vi "Compute Deconvolved IRF Plot.vi"(4 "# Fit Plot Points":i32=65536, 6 "IRF*PSED fixed Parameters":T1={"order"=0, "T"=0.0, "Time Constant Array"=[], "{S_k, C_k, phi_k, e_k} arrays"={"S_k Array"=[], "C_k Array"=[], "phi_k Array"=[], "e_k Array"=[]}, "IRF Extraction Options"={"Time Constant for IRF Extraction"=1e-18, "IRF Order"=0, "Fourier Series Smoothing"=enum."None", "Noise Threshold"=0.0, "Smoothing Width"=0.0, "Fourier Series Truncation"=enum."Automatic", "Truncation Order"=0, "Save Power Spectrum"=FALSE, "Smoothing"=FALSE, "Smoothing Parameter"=0.0, "Smoothing Order"=1, "Method"=enum."Direct"}} {"IRF Extraction Options"."Smoothing Order" min=1 max=10; "IRF Extraction Options"."Time Constant for IRF Extraction" format="%#_5g"}, 7 "XYGraph in":T6, 8 "error in (no error)":errorcluster, 9 "Fit Parameter Values":dbl[](array[numeric]), 10 "Plot Name":string, 11 "Fitted Decay":cluster{"X Array":dbl[], "Y Array":dbl[]}) -> (0 "error out":errorcluster, 1 "Amplitude String":string, 2 "Power Spectrum":dbl[](array[numeric]), 3 "IRF Plot":cluster{"X Array":dbl[], "Y Array":dbl[]}, 5 "Smoothed Power Spectrum":dbl[](array[numeric]))   [LabVIEW 2021, in "Fits.lvlib"]
uses:
  Fits.lvlib
  Graphs/XY Graph/XY Graph Refnum.ctl
  IRF(X)PSED Fixed Parameters v3.ctl
  IRF(X)PSED Extraction Options.ctl
  Fourier Series Smoothing Option.ctl
  Fourier Series Truncation.ctl
  IRF Extraction Method.ctl
  908e9038-7821-4251-955b-b37bdb3470f5.vi
  IRF Options.vi
  Graphs/XY Graph/XY Graph Add Single Plot with Name.vi
  Graphs/XY Graph/XY Graph Add-Ons.lvlib
  Arrays/Arrays.lvlib
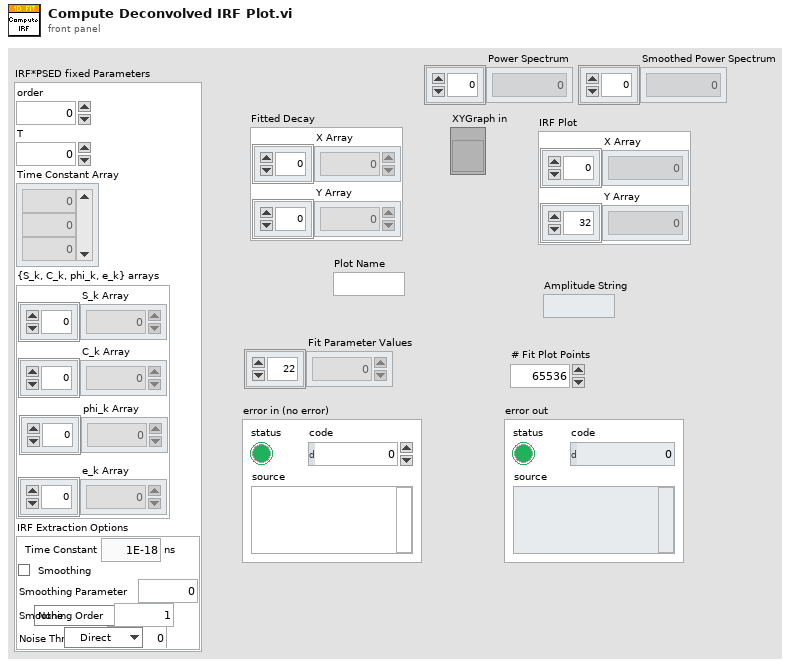
[diagram p1: front panel]
types:
  T1 = typedef "Fits.lvlib/IRF(X)PSED Fixed Parameters v3.ctl" = cluster{"order":i32, "T":dbl, "Time Constant Array":dbl[], "{S_k, C_k, phi_k, e_k} arrays":cluster{"S_k Array":dbl[], "C_k Array":dbl[], "phi_k Array":dbl[], "e_k Array":dbl[]}, "IRF Extraction Options":T2}
  T2 = typedef "Fits.lvlib/IRF(X)PSED Extraction Options.ctl" = cluster{"Time Constant for IRF Extraction":dbl[unit], "IRF Order":i32, "Fourier Series Smoothing":T3, "Noise Threshold":dbl, "Smoothing Width":dbl, "Fourier Series Truncation":T4, "Truncation Order":i32, "Save Power Spectrum":bool, "Smoothing":bool, "Smoothing Parameter":dbl, "Smoothing Order":u32, "Method":T5}
  T3 = typedef "Fits.lvlib/Fourier Series Smoothing Option.ctl" = enum16{"None", "Lanczos Factors", "Fejer Summation"}
  T4 = typedef "Fits.lvlib/Fourier Series Truncation.ctl" = enum16{"Automatic", "Fixed"}
  T5 = typedef "Fits.lvlib/IRF Extraction Method.ctl" = enum16{"Direct", "Topless", "Toeplitz"}
  T6 = typedef "XY Graph Add-Ons.lvlib/XY Graph Refnum.ctl" = refnum<vi>
  T7 = enum16{"Sum of Exponentials", "Squared Sum of Exponentials", "Fourier Series"}
  T8 = typedef "XY Graph Add-Ons.lvlib/XY Plot Data.ctl" = cluster{"X Array":dbl[], "Y Array":dbl[]}
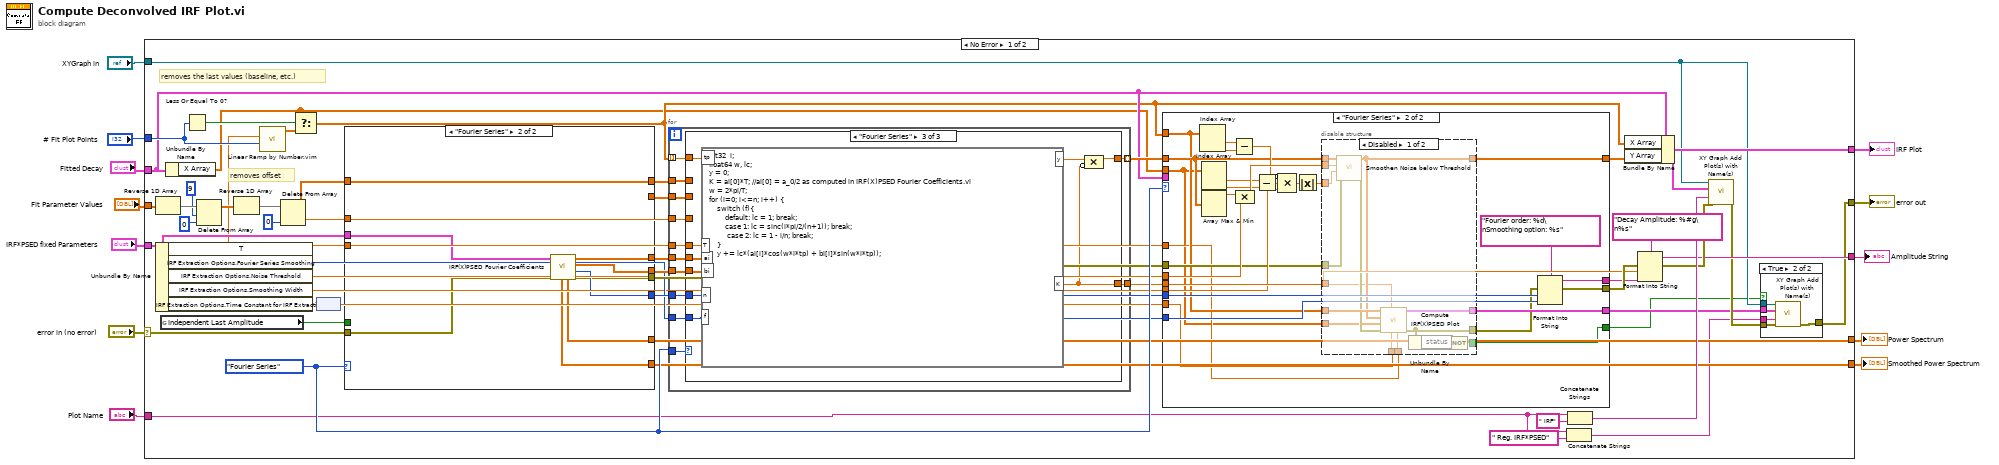
[diagram p0: block diagram]
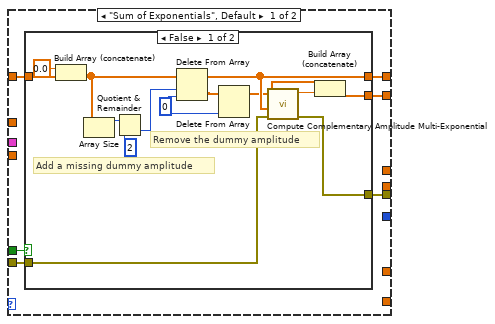
[diagram p5: hidden frame]
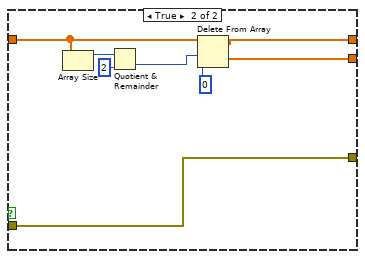
[diagram p6: hidden frame]
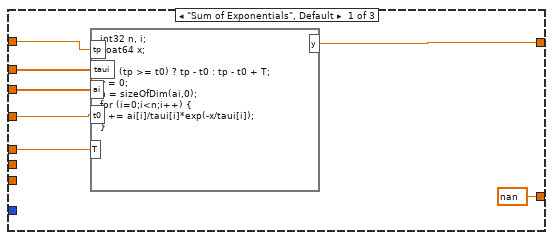
[diagram p7: hidden frame]
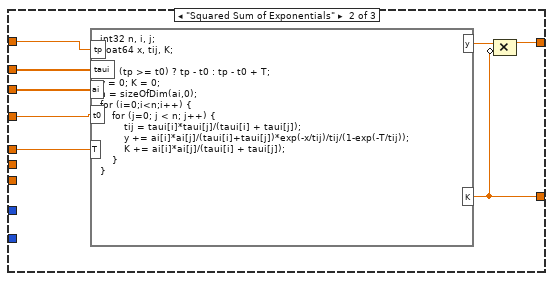
[diagram p8: hidden frame]
diagram:
  n1 = case shown="No Error" "error in (no error)" {
    selector: "error in (no error)" -> [w34 w191]
    tunnel: "Fit Parameter Values" -> [w60 _]
    tunnel: "Fitted Decay" -> [w37 _]
    tunnel: [w63 _] -> w10
    tunnel: "XYGraph in" -> [w21 _]
    tunnel: [w19 w191] -> w8
    tunnel: "IRF*PSED fixed Parameters" -> [w44 _]
    tunnel: "Plot Name" -> [w16 _]
    tunnel: "# Fit Plot Points" -> [w52 _]
    tunnel: [w48 _] -> w4
    tunnel: [w27 _] -> w2
    tunnel: [w26 _] -> w1
    frame No Error {
      w40 = T7."Fourier Series" ("IRF Model")
      # "removes offset"
      # "removes the last values (baseline, etc.)"
      n2 = Reverse 1D Array(array=w60) -> (reversed array=w59:dbl[])
      n3 = Unbundle By Name(w44) -> ("T"=w23:dbl, "IRF Extraction Options.Fourier Series Smoothing"=w30:T3, "IRF Extraction Options.Noise Threshold"=w28:dbl, "IRF Extraction Options.Smoothing Width"=w29:dbl, "IRF Extraction Options.Time Constant for IRF Extraction"=w24:dbl[unit])
      n4 = global read "IRF Options.vi" "Independent Last Amplitude"() -> (w45:bool)
      n5 = Unbundle By Name(w37) -> ("X Array"=w25:dbl[])
      n6 = Less Or Equal To 0?(x=w52) -> (x <= 0?=w53:bool)
      n7 = Delete From Array(array=w59, length=9, index=0) -> (array with subset deleted=w58:dbl[])  [unwired: 1 out]
      n8 = Reverse 1D Array(array=w58) -> (reversed array=w55:dbl[])
      n9 = call "Linear Ramp by Number.vim"("# Steps (1)"=w52, "End (1)"=w23) -> ("Ramp"=w51:dbl[])  [unwired: 7 in, 2 out]
      n10 = Delete From Array(array=w55, index=0) -> (deleted portion=w43:dbl, array with subset deleted=w54:dbl[])  [unwired: 1 in]
      n11 = Select(t=w25, s=w53, f=w51) -> (s? t:f=w36:dbl[])
      n12 = node(w24) -> (w22:dbl)
      n13 = case shown="\"Fourier Series\"" w40 {
        tunnel: w54 -> [w123 w154]
        tunnel: [w122 w154] -> w47
        tunnel: [w121 _] -> w46
        tunnel: w45 -> [w120 _]
        tunnel: w44 -> [_ w151]
        tunnel: w43 -> [_ _]
        tunnel: w23 -> [_ _]
        tunnel: [_ w153] -> w42
        tunnel: [_ w152] -> w41
        tunnel: [_ w150] -> w35
        tunnel: w34 -> [w119 w149]
        tunnel: [w118 w148] -> w33
        tunnel: [_ w147] -> w27
        tunnel: [_ w146] -> w26
        frame "Sum of Exponentials", Default {
          n14 = case shown="False" w120 {
            tunnel: w123 -> [w137 w141]
            tunnel: [w133 w140] -> w122
            tunnel: [w130 w139] -> w121
            tunnel: w119 -> [w125 w138]
            tunnel: [w124 w138] -> w118
            frame False {
              w134 = 0 ("index")
              # "Remove the dummy amplitude"
              # "Add a missing dummy amplitude"
              n15 = Build Array (concatenate)(0.0 ("element"), w137) -> (w127:dbl[])
              n16 = Array Size(array=w127) -> (size(s)=w128:i32)
              n17 = Quotient & Remainder(x=w128, y=2) -> (floor(x/y)=w126:i32)  [unwired: 1 out]
              n18 = Delete From Array(array=w127, length=w126, index=w134) -> (deleted portion=w135:dbl[], array with subset deleted=w133:dbl[])
              n19 = Delete From Array(array=w135, index=w134) -> (array with subset deleted=w132:dbl[])  [unwired: 1 in, 1 out]
              n20 = call "Compute Complementary Amplitude Multi-Exponential.vi"("Error In"=w125, "Time Constant Array"=w133, "Amplitude Array"=w132) -> ("Error Out"=w124:errorcluster, "Complementary Amplitude"=w131:dbl)  [unwired: 7 in]
              n21 = Build Array (concatenate)(w132, w131) -> (w130:dbl[])
            }
            frame True {
              n22 = Array Size(array=w141) -> (size(s)=w143:i32)
              n23 = Quotient & Remainder(x=w143, y=2) -> (floor(x/y)=w142:i32)  [unwired: 1 out]
              n24 = Delete From Array(array=w141, length=w142, index=0) -> (deleted portion=w139:dbl[], array with subset deleted=w140:dbl[])
            }
          }
        }
        frame "Fourier Series" {
          n25 = call "IRF(X)PSED Fourier Coefficients.vi"("Error In"=w149, "IRF*PSED fixed Parameters"=w151) -> ("Error Out"=w148:errorcluster, "Optimal Order"=w150:i32, "[b_k]"=w152:dbl[], "[a_k]"=w153:dbl[], "[s_k]"=w147:dbl[], "Smoothed [s_k]"=w146:dbl[])  [unwired: 4 in]
        }
      }
      n26 = for {
        tunnel: w36 -> [w166] mode=indexing
        tunnel: w43 -> [w165]
        tunnel: w46 -> [w164]
        tunnel: w47 -> [w163]
        tunnel: [w162] -> w39 mode=indexing
        tunnel: w23 -> [w161]
        tunnel: [w160] -> w13
        tunnel: w40 -> [w159]
        tunnel: w42 -> [w158]
        tunnel: w41 -> [w157]
        tunnel: w30 -> [w155]
        tunnel: w35 -> [w156]
        n27 = case shown="\"Fourier Series\"" w159 {
          tunnel: w166 -> [w173 w181 w190]
          tunnel: w165 -> [w172 w180 _]
          tunnel: w164 -> [w171 w179 _]
          tunnel: w163 -> [w170 w178 _]
          tunnel: [w169 w175 w187] -> w162
          tunnel: w161 -> [w168 w176 w188]
          tunnel: [nan ("K") w174 w186] -> w160
          tunnel: w158 -> [_ _ w185]
          tunnel: w157 -> [_ _ w182]
          tunnel: w156 -> [_ _ w184]
          tunnel: w155 -> [_ _ w183]
          frame "Sum of Exponentials", Default {
            n28 = formula code="int32 n, i;\nfloat64 x;\n\nx = (tp >= t0) ? tp - t0 : tp - t0 + T;\ny = 0;\nn = sizeOfDim(ai,0);\nfor (i=0;i<n;i++) {\ny += ai[i]/taui[i]*exp(-x/taui[i]);\n}"("tp"=w173, "t0"=w172, "ai"=w171, "taui"=w170, "T"=w168) -> ("y"=w169:dbl)
          }
          frame "Squared Sum of Exponentials" {
            n29 = formula code="int32 n, i, j;\nfloat64 x, tij, K;\n\nx = (tp >= t0) ? tp - t0 : tp - t0 + T;\ny = 0; K = 0;\nn = sizeOfDim(ai,0);\nfor (i=0;i<n;i++) {\n    for (j=0; j < n; j++) {\n        tij = taui[i]*taui[j]/(taui[i] + taui[j]);\n        y += ai[i]*ai[j]/(taui[i]+taui[j])*exp(-x/tij)/tij/(1-exp(-T/tij));\n        K += ai[i]*ai[j]/(taui[i] + taui[j]);\n    }\n}"("tp"=w181, "t0"=w180, "ai"=w179, "taui"=w178, "T"=w176) -> ("y"=w177:dbl, "K"=w174:dbl)
            n30 = Compound Arithmetic op=MULTIPLY(w177, invert w174) -> (w175:dbl)
          }
          frame "Fourier Series" {
            n31 = formula code="int32  i;\nfloat64 w, lc;\ny = 0;\nK = ai[0]*T; //ai[0] = a_0/2 as computed in IRF(X)PSED Fourier Coefficients.vi \nw = 2*pi/T;\nfor (i=0; i<=n; i++) {\n    switch (f){\n        default: lc = 1; break; \n        case 1: lc = sinc(i*pi/2/(n+1)); break;\n         case 2: lc = 1 - i/n; break;\n    }\n    y += lc*(ai[i]*cos(w*i*tp) + bi[i]*sin(w*i*tp));\n}"("tp"=w190, "ai"=w185, "T"=w188, "bi"=w182, "n"=w184, "f"=w183) -> ("y"=w189:dbl, "K"=w186:dbl)
            n32 = Compound Arithmetic op=MULTIPLY(w189, invert w186) -> (w187:dbl)
          }
        }
      }
      n33 = case shown="\"Fourier Series\"" w40 {
        tunnel: w39 -> [w72 w83]
        tunnel: [w72 w80] -> w38
        tunnel: w37 -> [_ _]
        tunnel: w36 -> [_ w81]
        tunnel: w28 -> [_ w100]
        tunnel: w29 -> [_ w97]
        tunnel: w25 -> [_ w77]
        tunnel: w30 -> [_ w87]
        tunnel: w35 -> [_ w86]
        tunnel: w33 -> [w71 w82]
        tunnel: [w71 w85] -> w32
        tunnel: [_ w84] -> w31
        tunnel: w22 -> [_ w79]
        tunnel: w23 -> [_ w78]
        tunnel: [_ w76] -> w18
        tunnel: [_ w73] -> w17
        tunnel: w13 -> [_ w74]
        frame "Sum of Exponentials", Default {
        }
        frame "Fourier Series" {
          n34 = Index Array(array=w81) -> (element #1=w96:dbl, element #2=w95:dbl)  [unwired: 2 in]
          n35 = Index Array(array=w77) -> (element #1=w94:dbl, element #2=w93:dbl)  [unwired: 2 in]
          n36 = Array Max & Min(array=w83) -> (max value=w98:dbl)  [unwired: 3 out]
          n37 = Subtract(x=w96, y=w95) -> (x-y=w92:dbl)
          n38 = Compound Arithmetic op=MULTIPLY(w98, w100) -> (w99:dbl)
          n39 = Subtract(x=w94, y=w93) -> (x-y=w91:dbl)
          n40 = Compound Arithmetic op=MULTIPLY(invert w92, w91, w97) -> (w90:dbl)
          n41 = Absolute Value(x=w90) -> (abs(x)=w89:dbl)
          n42 = disable-structure shown="Disabled" {
            disable-tunnel: w99 -> [w115 _]
            disable-tunnel: w89 -> [w114 _]
            disable-tunnel: w83 -> [w113 w117]
            disable-tunnel: w82 -> [w112 w116]
            disable-tunnel: w81 -> [w111 _]
            disable-tunnel: [w110 w117] -> w80
            disable-tunnel: w79 -> [w108 _]
            disable-tunnel: w78 -> [w107 _]
            disable-tunnel: w77 -> [w106 _]
            disable-tunnel: [w105 _] -> w76
            disable-tunnel: [w104 w116] -> w75
            disable-tunnel: w74 -> [w103 _]
            disable-tunnel: [w101 _] -> w73
            frame Disabled {
              n43 = call "Smoothen Noise below Threshold.vi"("Error In"=w112, "Smoothing Width"=w114, "Noise Threshold"=w115, "Function in"=w113) -> ("Error Out"=w109:errorcluster, "Function out"=w110:dbl[])  [unwired: 6 in]
              n44 = call "Compute IRF(X)PSED Plot.vi"("Period T"=w107, "Lifetime tau"=w108, "Prefactor"=w103, "error in (no error)"=w109, "Decay X array"=w106, "IRF Y Array"=w110, "IRF X array"=w111) -> ("error out"=w104:errorcluster, "IRF*PSED Plot"=w105:T8)  [unwired: 3 in]
              n45 = Unbundle By Name(w104) -> ("status"=w102:bool)
              n46 = Not(x=w102) -> (.not. x?=w101:bool)
            }
            frame Enabled {
            }
          }
          n47 = Format Into String(format string="Fourier order: %d\nSmoothing option: %s", error in=w75, w86, w87) -> (resulting string=w84:string, error out=w85:errorcluster)  [unwired: 1 in]
        }
      }
      n48 = Concatenate Strings(w16, " Reg. IRF*PSED" ("string")) -> (w15:string)
      n49 = Concatenate Strings(w16, " IRF" ("string")) -> (w61:string)
      n50 = Bundle By Name(cluster=w37, "X Array"=w36, "Y Array"=w38) -> (w63:cluster{"X Array":dbl[], "Y Array":dbl[]})
      n51 = Format Into String(format string="Decay Amplitude: %#g\n%s", error in=w32, w13, w31) -> (resulting string=w48:string, error out=w49:errorcluster)  [unwired: 1 in]
      n52 = call-poly "XY Graph Add Plot(s) with Name(s).vi"("XYGraph Ref in"=w21, "Plot"=w63, "Plot Name (\"Plot\")"=w61, "error in (no error)"=w49) -> ("error out"=w20:errorcluster)  [unwired: 8 in, 3 out]
      n53 = case shown="True" w17 {
        tunnel: w21 -> [_ w70]
        tunnel: w20 -> [w65 w69]
        tunnel: [w65 w68] -> w19
        tunnel: w18 -> [_ w67]
        tunnel: w15 -> [_ w66]
        frame False {
        }
        frame True {
          n54 = call-poly "XY Graph Add Plot(s) with Name(s).vi"("XYGraph Ref in"=w70, "Plot"=w67, "Plot Name (\"Plot\")"=w66, "error in (no error)"=w69) -> ("error out"=w68:errorcluster)  [unwired: 8 in, 3 out]
        }
      }
    }
    frame Error {
    }
  }
  "IRF Plot" <- w10
  "error out" <- w8
  "Amplitude String" <- w4
  "Power Spectrum" <- w2
  "Smoothed Power Spectrum" <- w1
